vi "Read Serial Data.vi"(8 "error in (no error)":errorcluster, 11 "VISA Refnum in":refnum<visa-resource-name>) -> (0 "error out":errorcluster, 1 "Analog Inputs":T1, 2 "Switch Inputs":T2, 3 "VISA Refnum out":refnum<visa-resource-name>, 4 "CRC Status":bool)   [LabVIEW 2013]
uses:
  Switch_Input_TypeDef.ctl
  Analog_Input_TypeDef.ctl
  Inline CRC/CRC SubVIs/Wrappers/CRC-8-Maxim 1-Wire (DOW).vi
  <vilib>/Utility/error.llb/Error Cluster From Error Code.vi
  <vilib>/ErrorRing/Error Ring.xnode
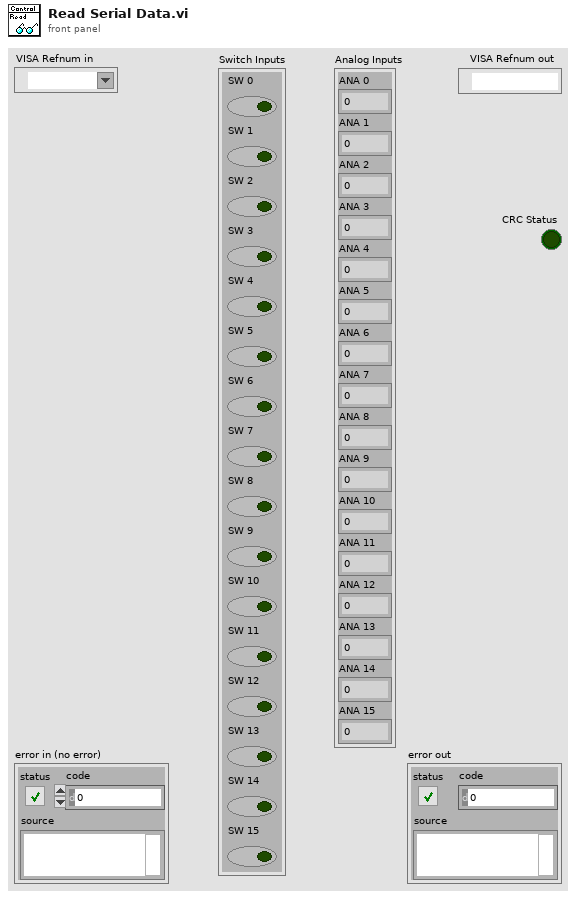
[diagram p1: front panel]
types:
  T1 = typedef "Analog_Input_TypeDef.ctl" = cluster{"ANA 0":u8, "ANA 1":u8, "ANA 2":u8, "ANA 3":u8, "ANA 4":u8, "ANA 5":u8, "ANA 6":u8, "ANA 7":u8, "ANA 8":u8, "ANA 9":u8, "ANA 10":u8, "ANA 11":u8, "ANA 12":u8, "ANA 13":u8, "ANA 14":u8, "ANA 15":u8}
  T2 = typedef "Switch_Input_TypeDef.ctl" = cluster{"SW 0":bool, "SW 1":bool, "SW 2":bool, "SW 3":bool, "SW 4":bool, "SW 5":bool, "SW 6":bool, "SW 7":bool, "SW 8":bool, "SW 9":bool, "SW 10":bool, "SW 11":bool, "SW 12":bool, "SW 13":bool, "SW 14":bool, "SW 15":bool}
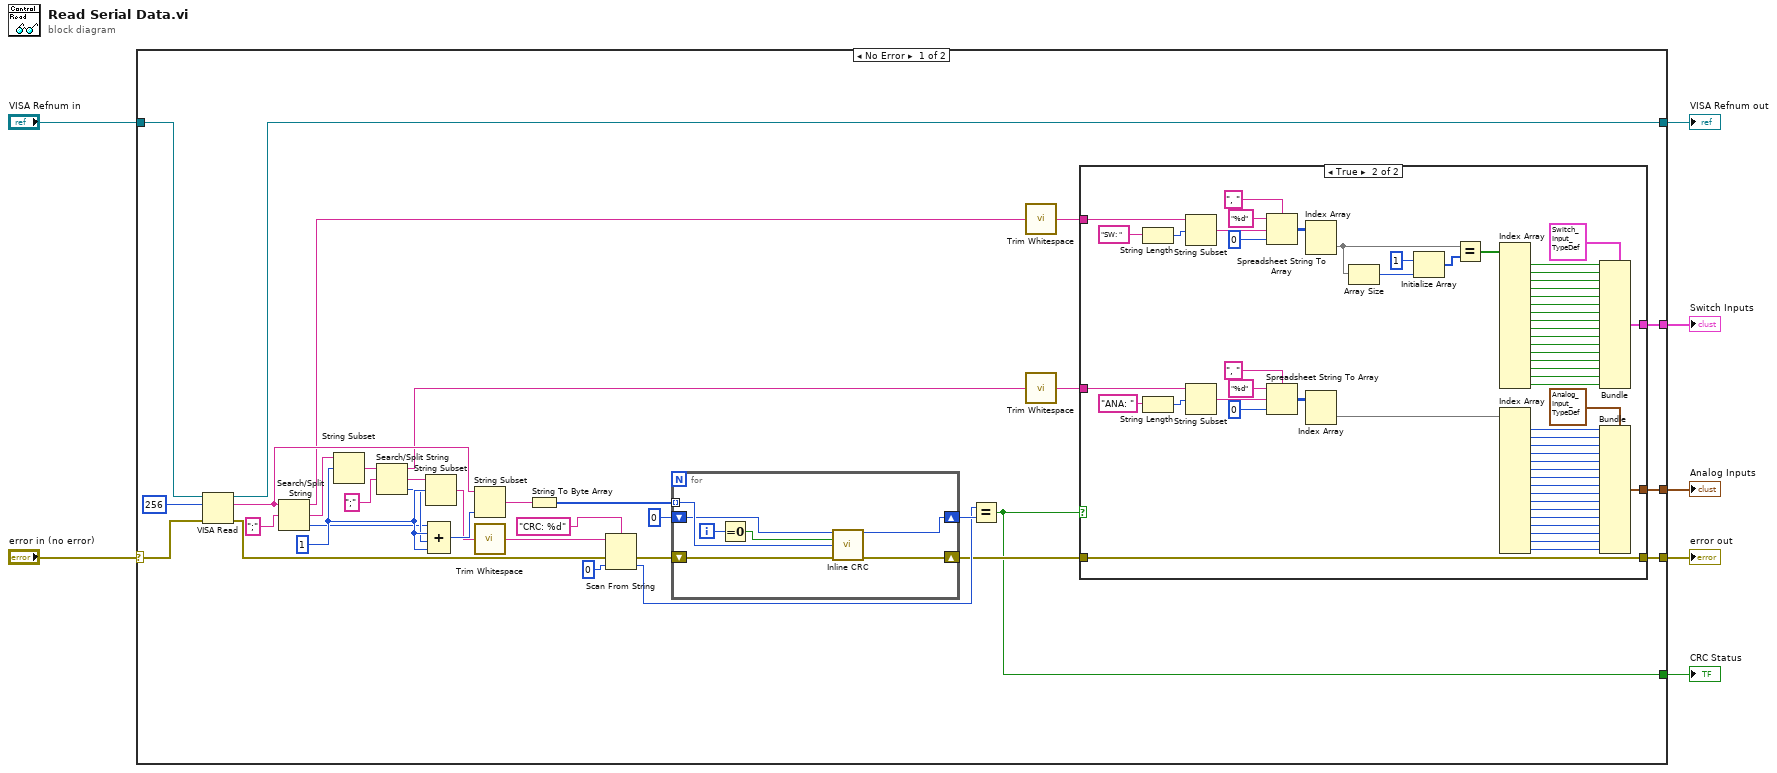
[diagram p0: block diagram]
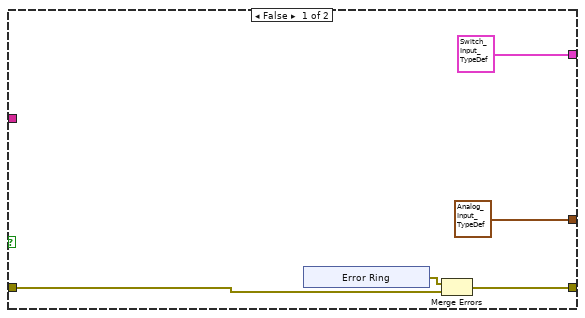
[diagram p2: hidden frame]
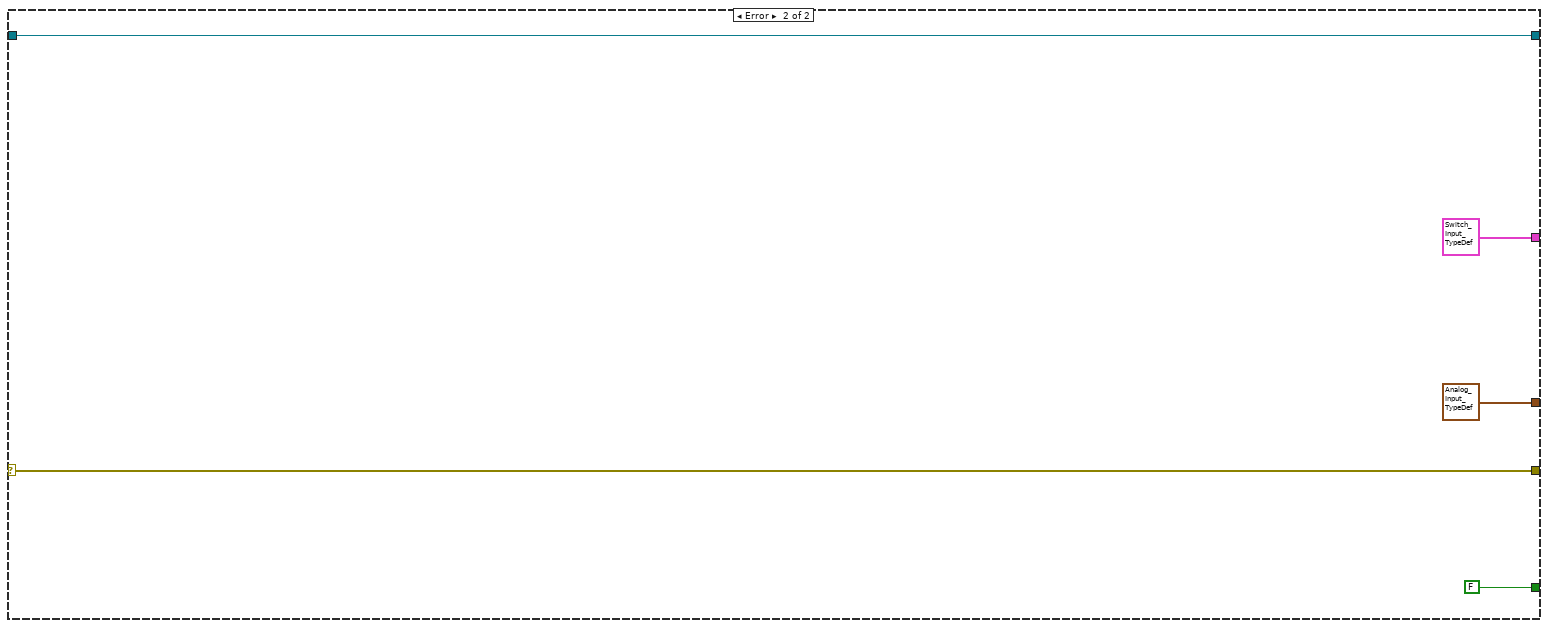
[diagram p3: hidden frame]
diagram:
  n1 = case shown="No Error" "error in (no error)" {
    selector: "error in (no error)" -> [w10 w121]
    tunnel: [w21 w122] -> w7
    tunnel: "VISA Refnum in" -> [w19 w122]
    tunnel: [w17 T2 {"SW 0"=FALSE, "SW 1"=FALSE, "SW 2"=FALSE, "SW 3"=FALSE, "SW 4"=FALSE, "SW 5"=FALSE, "SW 6"=FALSE, "SW 7"=FALSE, "SW 8"=FALSE, "SW 9"=FALSE, "SW 10"=FALSE, "SW 11"=FALSE, "SW 12"=FALSE, "SW 13"=FALSE, "SW 14"=FALSE, "SW 15"=FALSE} ("Switch Inputs")] -> w5
    tunnel: [w14 w121] -> w4
    tunnel: [w13 T1 {"ANA 0"=0, "ANA 1"=0, "ANA 2"=0, "ANA 3"=0, "ANA 4"=0, "ANA 5"=0, "ANA 6"=0, "ANA 7"=0, "ANA 8"=0, "ANA 9"=0, "ANA 10"=0, "ANA 11"=0, "ANA 12"=0, "ANA 13"=0, "ANA 14"=0, "ANA 15"=0} ("Analog Inputs")] -> w3
    tunnel: [w9 FALSE] -> w1
    frame No Error {
      w31 = 1 ("offset (0)")
      n2 = VISA Read(VISA resource name=w19, byte count=u32 256, error in (no error)=w10) -> (VISA resource name out=w21:refnum<visa-resource-name>, read buffer=w32:string, error out=w12:errorcluster)  [unwired: 1 out]
      n3 = Search/Split String(string=w32, search string/char (-)=";") -> (substring before match=w24:string, match + rest of string=w27:string, offset of match=w29:i32)  [unwired: 1 in]
      n4 = String Subset(string=w27, offset (0)=w31) -> (substring=w28:string)  [unwired: 1 in]
      n5 = Search/Split String(string=w28, search string/char (-)=";") -> (substring before match=w23:string, match + rest of string=w25:string, offset of match=w30:i32)  [unwired: 1 in]
      n6 = String Subset(string=w25, offset (0)=w31) -> (substring=w26:string)  [unwired: 1 in]
      n7 = Compound Arithmetic op=ADD(w29, w31, w30, w31) -> (w33:i32)
      n8 = String Subset(string=w32, length (rest)=w33) -> (substring=w34:string)  [unwired: 1 in]
      n9 = call <vilib>:"Trim Whitespace.vi"("string"=w26) -> ("trimmed string"=w37:string)  [unwired: 1 in]
      n10 = String To Byte Array(string=w34) -> (unsigned byte array=w35:u8[])
      n11 = Scan From String(format string="CRC: %d", input string=w37, error in=w12, default 1=u8 0 ("CRC")) -> (error out=w11:errorcluster, output 1=w39:u8)  [unwired: 1 in, 2 out]
      n12 = for {
        tunnel: w35 -> [w117] mode=indexing
        shift-right: [w115] -> w40
        shift-left: u8 0 ("CRC") -> [w116]
        shift-right: [w111] -> w15
        shift-left: w11 -> [w112]
        i -> [w114]
        n13 = Equal To 0?(x=w114) -> (x = 0?=w113:bool)
        n14 = call-poly "Inline CRC.vi"("CRC In"=w116, "Reset"=w113, "Data"=w117, "error in (no error)"=w112) -> ("CRC"=w115:u8, "error out"=w111:errorcluster)  [unwired: 10 in]
      }
      n15 = Equal?(x=w39, y=w40) -> (x = y?=w9:bool)
      n16 = call <vilib>:"Trim Whitespace.vi"("string"=w24) -> ("trimmed string"=w18:string)  [unwired: 1 in]
      n17 = call <vilib>:"Trim Whitespace.vi"("string"=w23) -> ("trimmed string"=w16:string)  [unwired: 1 in]
      n18 = case shown="True" w9 {
        tunnel: w18 -> [_ w110]
        tunnel: [T2 {"SW 0"=FALSE, "SW 1"=FALSE, "SW 2"=FALSE, "SW 3"=FALSE, "SW 4"=FALSE, "SW 5"=FALSE, "SW 6"=FALSE, "SW 7"=FALSE, "SW 8"=FALSE, "SW 9"=FALSE, "SW 10"=FALSE, "SW 11"=FALSE, "SW 12"=FALSE, "SW 13"=FALSE, "SW 14"=FALSE, "SW 15"=FALSE} ("Switch Inputs") w90] -> w17
        tunnel: w16 -> [_ w70]
        tunnel: w15 -> [w42 w60]
        tunnel: [w44 w60] -> w14
        tunnel: [T1 {"ANA 0"=0, "ANA 1"=0, "ANA 2"=0, "ANA 3"=0, "ANA 4"=0, "ANA 5"=0, "ANA 6"=0, "ANA 7"=0, "ANA 8"=0, "ANA 9"=0, "ANA 10"=0, "ANA 11"=0, "ANA 12"=0, "ANA 13"=0, "ANA 14"=0, "ANA 15"=0} ("Analog Inputs") w69] -> w13
        frame False {
          n19 = xnode "Error Ring"() -> ("error out"=w43:errorcluster)
          n20 = Merge Errors(w43, w42) -> (w44:errorcluster)
        }
        frame True {
          n21 = String Length(string="SW: ") -> (length=w108:i32)
          n22 = String Length(string="ANA: ") -> (length=w72:i32)
          n23 = String Subset(string=w110, offset (0)=w108) -> (substring=w68:string)  [unwired: 1 in]
          n24 = String Subset(string=w70, offset (0)=w72) -> (substring=w58:string)  [unwired: 1 in]
          n25 = Spreadsheet String To Array(delimiter (Tab)=", ", format string="%d", spreadsheet string=w68, array type (2D Dbl)=u8 0) -> (array=w66:u8[][])
          n26 = Spreadsheet String To Array(delimiter (Tab)=", ", format string="%d", spreadsheet string=w58, array type (2D Dbl)=u8 0) -> (array=w57:u8[][])
          n27 = Index Array(array=w66) -> (element=w62:u8[])  [unwired: 2 in]
          n28 = Index Array(array=w57) -> (element=w56:u8[])  [unwired: 2 in]
          n29 = Array Size(array=w62) -> (size(s)=w61:i32)
          n30 = Initialize Array(u8 1, w61) -> (w64:u8[])
          n31 = Equal?(x=w62, y=w64) -> (x = y?=w65:bool[])
          n32 = Index Array(array=w65) -> (element #1=w106:bool, element #2=w105:bool, element #3=w91:bool, element #4=w92:bool, element #5=w93:bool, element #6=w94:bool, element #7=w95:bool, element #8=w96:bool, element #9=w97:bool, element #10=w98:bool, element #11=w99:bool, element #12=w100:bool, element #13=w101:bool, element #14=w102:bool, element #15=w103:bool, element #16=w104:bool)  [unwired: 16 in]
          n33 = Index Array(array=w56) -> (element #1=w74:u8, element #2=w75:u8, element #3=w89:u8, element #4=w88:u8, element #5=w87:u8, element #6=w86:u8, element #7=w85:u8, element #8=w84:u8, element #9=w83:u8, element #10=w82:u8, element #11=w81:u8, element #12=w80:u8, element #13=w79:u8, element #14=w78:u8, element #15=w77:u8, element #16=w76:u8)  [unwired: 16 in]
          n34 = Bundle(cluster=T2 {"SW 0"=FALSE, "SW 1"=FALSE, "SW 2"=FALSE, "SW 3"=FALSE, "SW 4"=FALSE, "SW 5"=FALSE, "SW 6"=FALSE, "SW 7"=FALSE, "SW 8"=FALSE, "SW 9"=FALSE, "SW 10"=FALSE, "SW 11"=FALSE, "SW 12"=FALSE, "SW 13"=FALSE, "SW 14"=FALSE, "SW 15"=FALSE} ("Switch Inputs"), "SW 0"=w106, "SW 1"=w105, "SW 2"=w91, "SW 3"=w92, "SW 4"=w93, "SW 5"=w94, "SW 6"=w95, "SW 7"=w96, "SW 8"=w97, "SW 9"=w98, "SW 10"=w99, "SW 11"=w100, "SW 12"=w101, "SW 13"=w102, "SW 14"=w103, "SW 15"=w104) -> (w90:T2)
          n35 = Bundle(cluster=T1 {"ANA 0"=0, "ANA 1"=0, "ANA 2"=0, "ANA 3"=0, "ANA 4"=0, "ANA 5"=0, "ANA 6"=0, "ANA 7"=0, "ANA 8"=0, "ANA 9"=0, "ANA 10"=0, "ANA 11"=0, "ANA 12"=0, "ANA 13"=0, "ANA 14"=0, "ANA 15"=0} ("Analog Inputs"), "ANA 0"=w74, "ANA 1"=w75, "ANA 2"=w89, "ANA 3"=w88, "ANA 4"=w87, "ANA 5"=w86, "ANA 6"=w85, "ANA 7"=w84, "ANA 8"=w83, "ANA 9"=w82, "ANA 10"=w81, "ANA 11"=w80, "ANA 12"=w79, "ANA 13"=w78, "ANA 14"=w77, "ANA 15"=w76) -> (w69:T1)
        }
      }
    }
    frame Error {
    }
  }
  "error out" <- w4
  "VISA Refnum out" <- w7
  "Switch Inputs" <- w5
  "Analog Inputs" <- w3
  "CRC Status" <- w1
